vi "Main.vi"() -> ()   [LabVIEW 2024]
uses:
  1. CTL/Brain_Loop_CTL.ctl
  <vilib>/Utility/miscctls.llb/LVPointTypeDef.ctl
  <vilib>/Utility/sysdir.llb/System Directory Type.ctl
panel:
  in  "Python 경로":path=path "D:/Python39-32/python.exe"
  in  "모듈 경로":path=path "C:/Users/user/Desktop/CATS_V3.0/5. Python/Generate_map.py"
  in  "Subscribe_모듈 경로":path=path "C:/Users/user/Desktop/CATS_V3.0/5. Python/Mqtt_Subscribe_Client.py"
  in  "Publish_모듈 경로_2":path=path "C:/Users/user/Desktop/CATS_V3.0/5. Python/Mqtt_Publish_Client.py"
  in  "Publish_모듈 경로":path=path "C:/Users/user/Desktop/CATS_V3.0/5. Python/Mqtt_Publish_Client.py"
  out "2_3_Station_Averange_SoundSpeed_Chart":dbl(graph)
  out "Water_Velocity_Chart":dbl(graph)
  in  "거리":dbl=3750.0 format="%#_13g"
  in  "유속 데이터":T1
  in  "데이터 통계":T2
  in  "관리자":T3
  out "TX_그래프 5":bool
  out "RX_그래프 5":bool
  out "TX_LED_4":bool
  out "RX_LED_4":bool
  out "TX_그래프":bool
  out "RX_그래프":bool
  out "Station_5":i32[](graph)
  out "Station_4":i32[](graph)
  out "Station_1":i32[](graph)
  out "C":dbl
  out "3_Station_Index":i32
  out "2_Station_Index":i32
  out "반환값":string
  in  "전체메뉴_탭_컨트롤":enum32{"지도", "데이터 통계", "관리자", "유속 데이터"}(tab)=enum."데이터 통계"
  out "Station_3_송신시작":string
  out "Station_2_송신시작":string
  out "Station_2":i32[](graph)
  out "Station_3":i32[](graph)
  out "TX_LED_2":bool
  out "RX_LED_2":bool
  out "TX_LED_3":bool
  out "RX_LED_3":bool
  in  "관리자_내부_탭_컨트롤":enum32{"실시간 현황", "Setting"}(tab) caption="탭 컨트롤 2"
  out "Station_현황_GPS":i32[](listbox)
  out "데이터 통계 현황_결과창":string
  out "Station_현황_TRX_Controller":i32[](listbox)
  out "적용_LED 2":bool
  in  "Wake_UP버튼":bool
  out "지도모듈_LED":bool
  in  "지도":T4
  in  "Order":i32=12
  in  "Q 값":i32=4
  out "적용_LED":bool
  in  "적용 버튼":bool
  in  "정지":bool
  out "시작일":string
  out "로그 기록":string
  out "2_3_Station_Averange_SoundSpeed":dbl
  out "Water_Velocity":dbl
  # "Costal Acoustic Tomography(Ver1.1)"
  # "데이터 통계 현황"
  # "Costal Acoustic Tomography Setting"
  # "Coastal_TMC_Set_Variable"
  # "Coastal_TMC_Map_Web"
  # "Sation_Wake_UP"
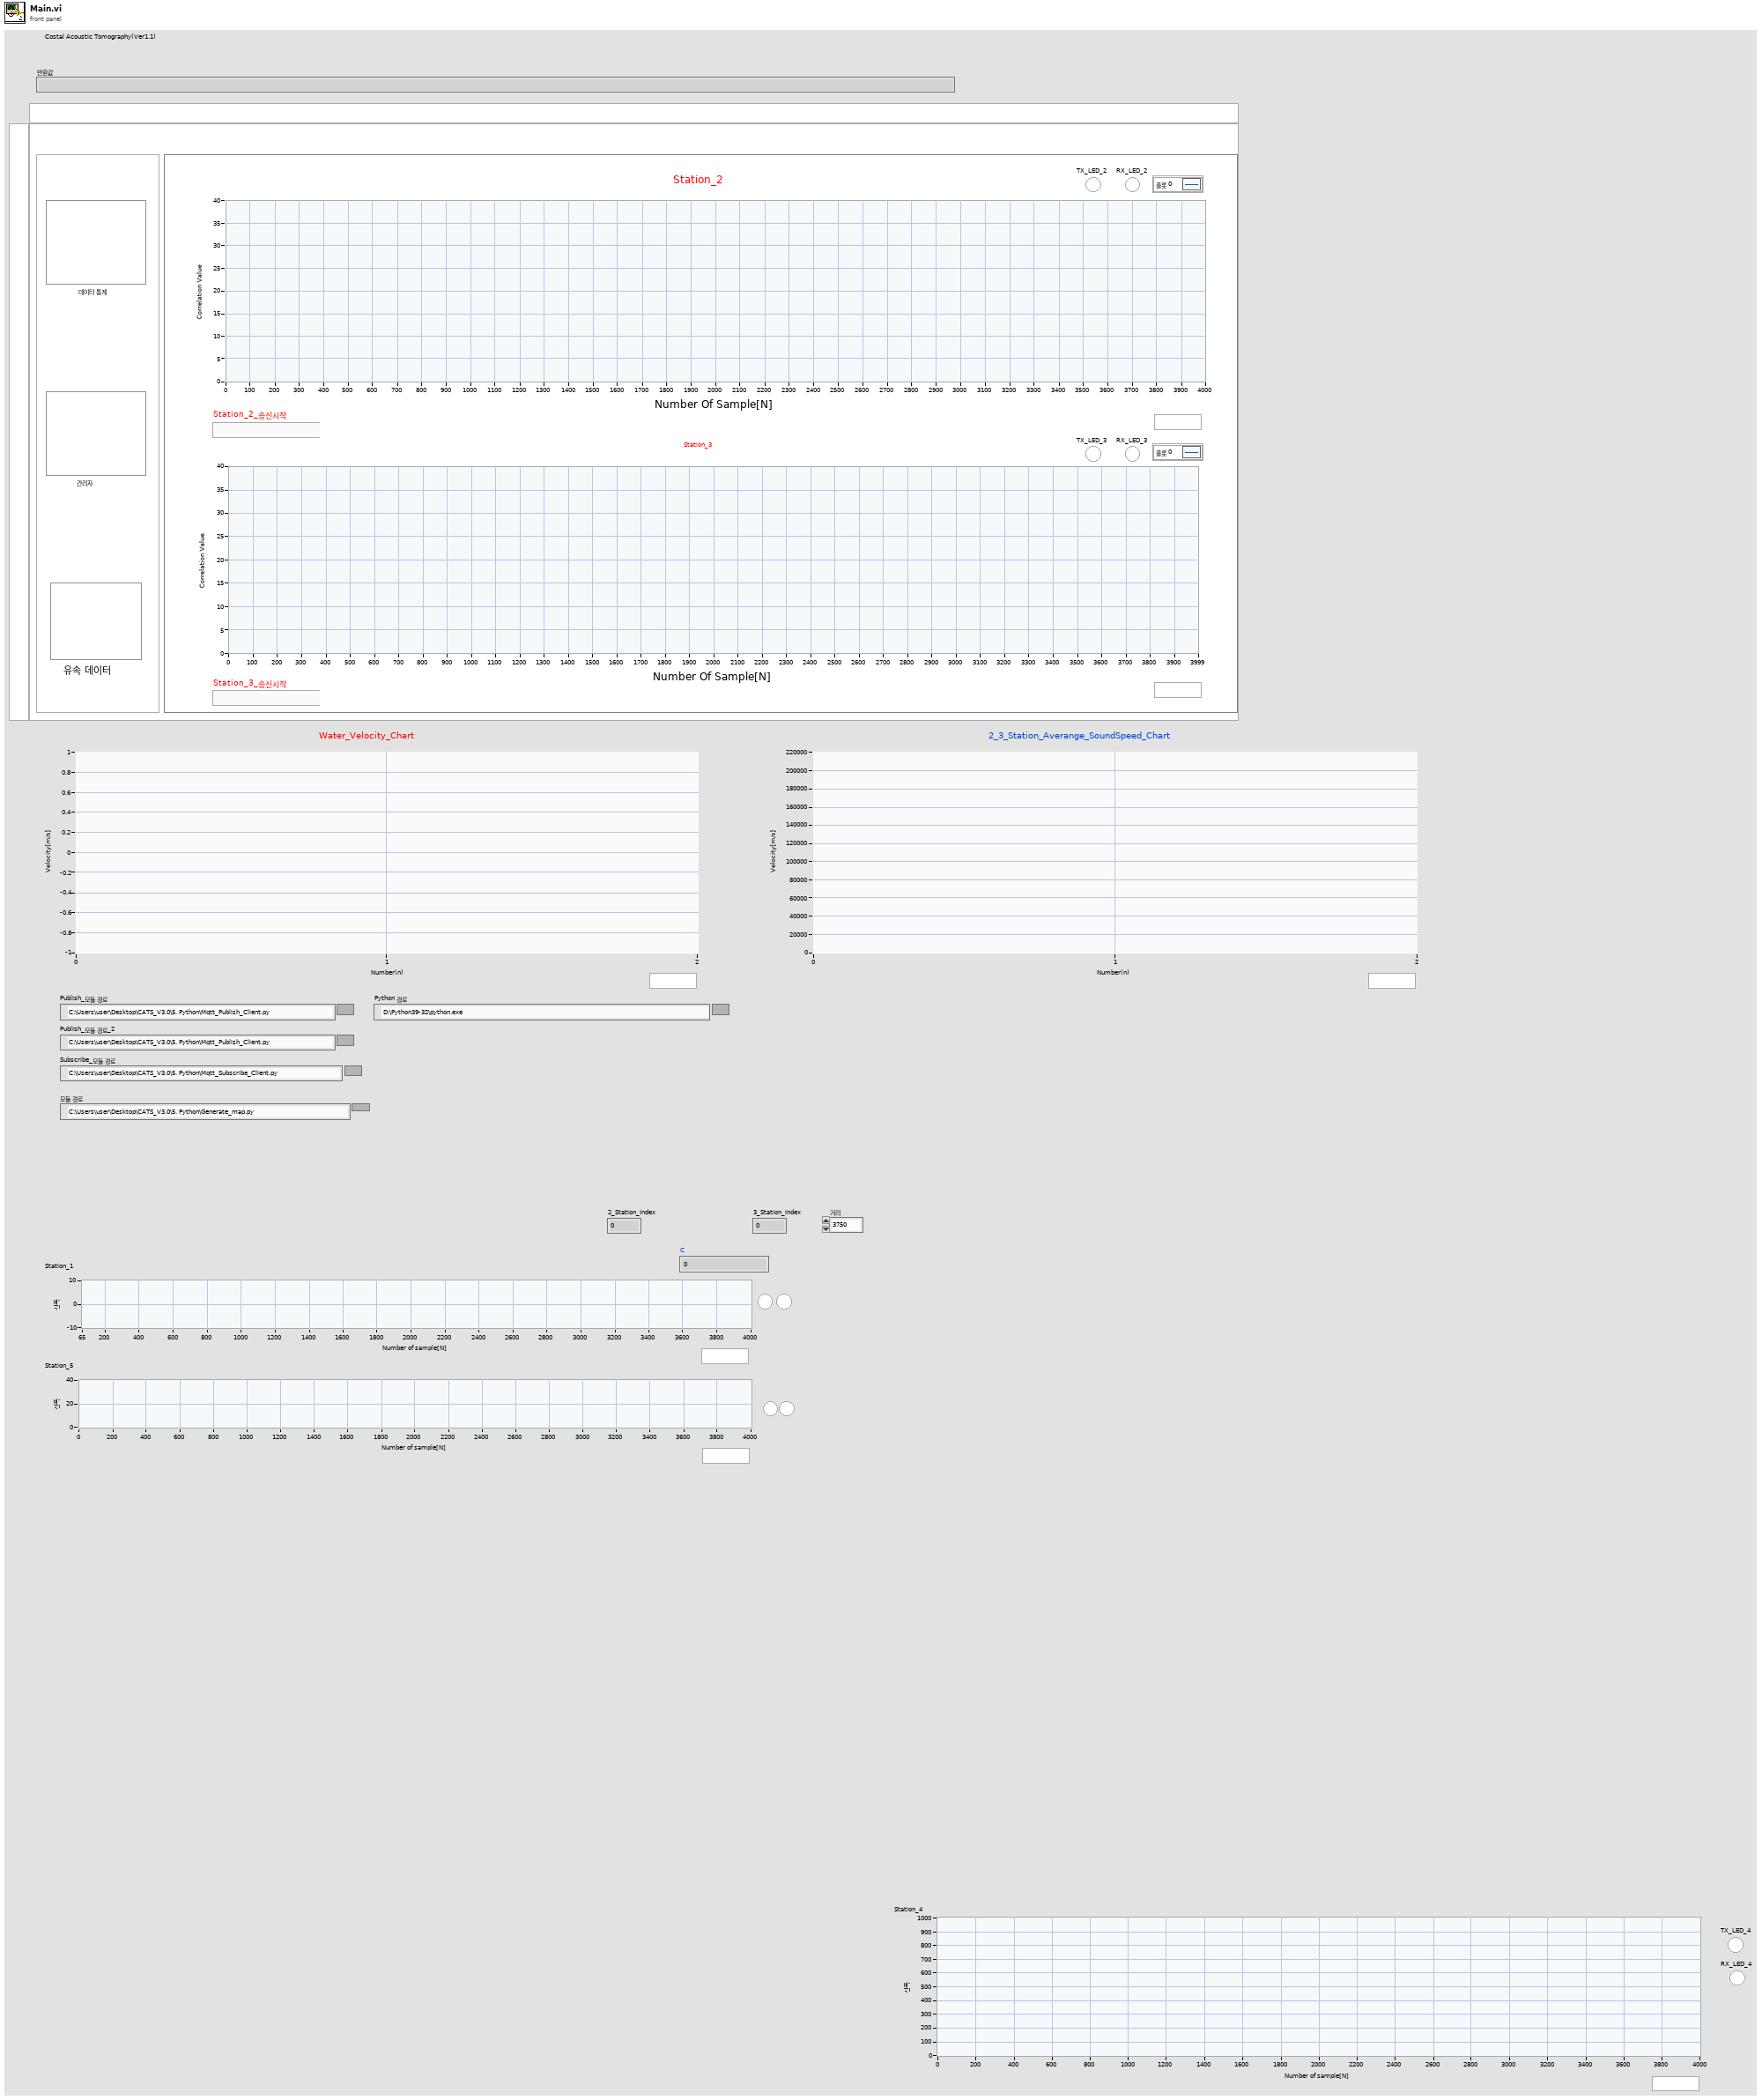
[diagram p1: front panel]
types:
  T1 = typedef "알림 컨트롤.ctl" = bool
  T2 = typedef "데이터 컨트롤.ctl" = bool
  T3 = typedef "관리 컨트롤.ctl" = bool
  T4 = typedef "지도 컨트롤.ctl" = bool
  T5 = cluster{"TX_그래프_LED":bool, "TX_그래프2_LED":bool, "TX_그래프3_LED":bool, "TX_그래프4_LED":bool, "TX_그래프5_LED":bool}
  T6 = cluster{"RX_그래프_LED":bool, "RX_그래프2_LED":bool, "RX_그래프3_LED":bool, "RX_그래프4_LED":bool, "RX_그래프5_LED":bool, "로그기록":string, "1_Station_Index":i32, "2_Station_Index":i32, "3_Station_Index":i32, "4_Station_Index":i32, "5_Station_Index":i32, "Velocity":dbl, "S_Flag":bool, "현재 날짜":string, "초기 날짜":string}
  T7 = typedef "Brain_Loop_CTL.ctl" = enum16{"초기화", "Mqtt_Subscribe", "Mqtt_Publish", "지도", "관리자", "데이터통계", "유속 데이터", "정지", "Mqtt_Publish_2"}
  T8 = typedef "LVPointTypeDef.ctl" = cluster{"Horizontal":i16, "Vertical":i16}
  T9 = typedef "System Directory Type.ctl" = i32
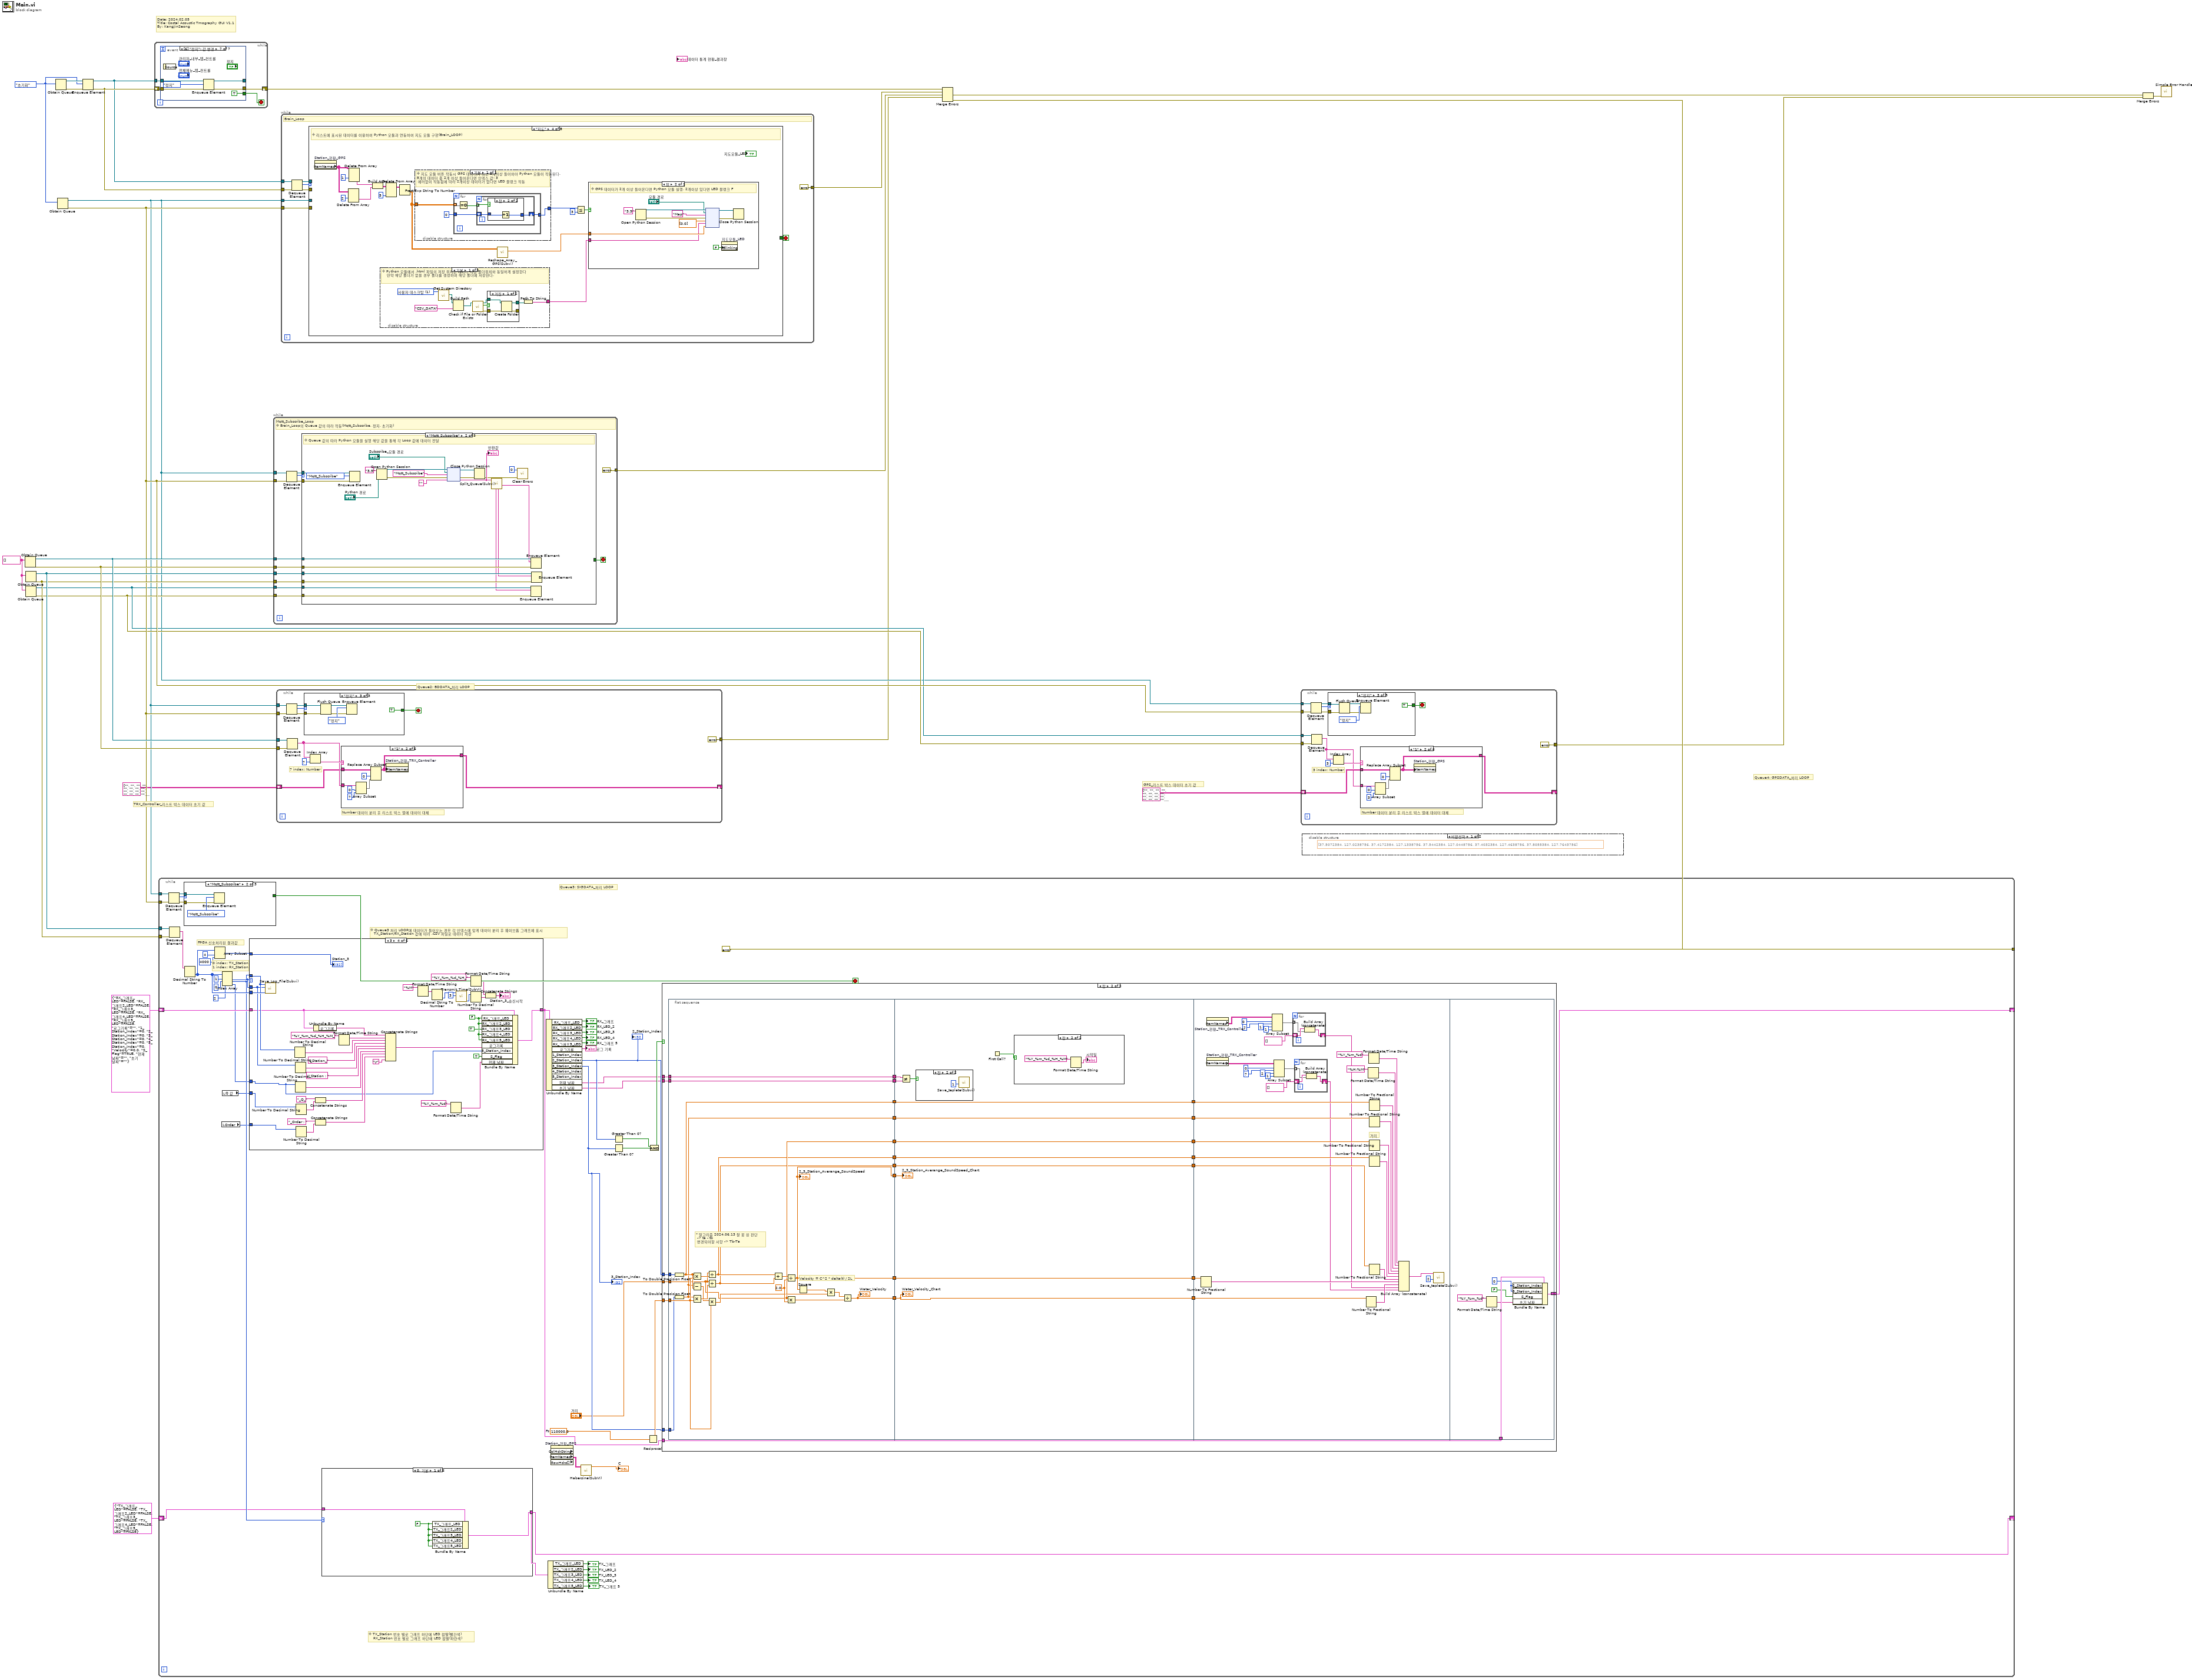
[diagram p0: block diagram]
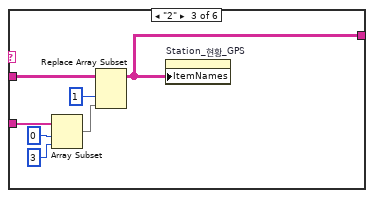
[diagram p4: hidden frame]
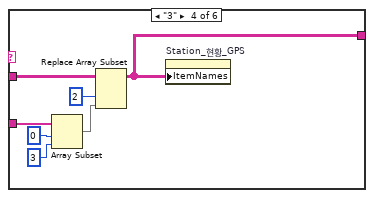
[diagram p5: hidden frame]
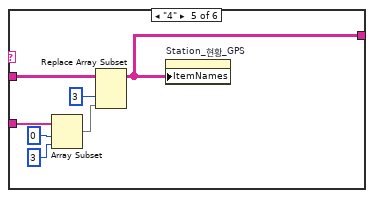
[diagram p6: hidden frame]
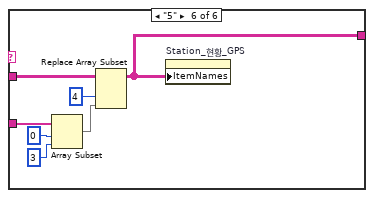
[diagram p7: hidden frame]
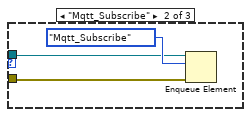
[diagram p9: hidden frame]
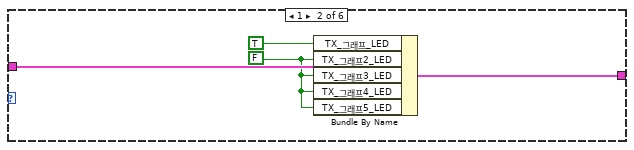
[diagram p13: hidden frame]
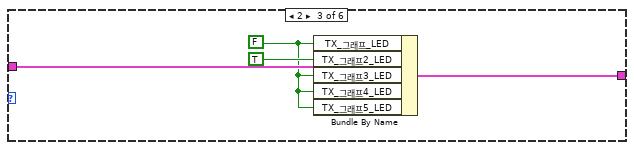
[diagram p14: hidden frame]
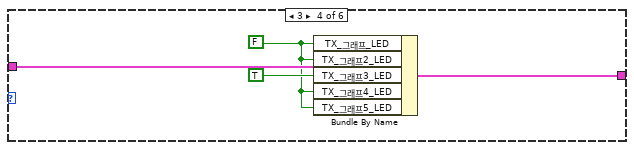
[diagram p15: hidden frame]
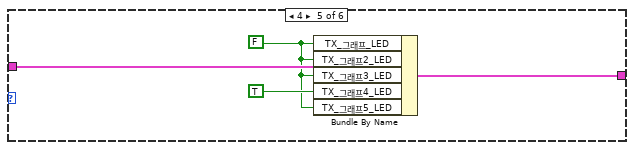
[diagram p16: hidden frame]
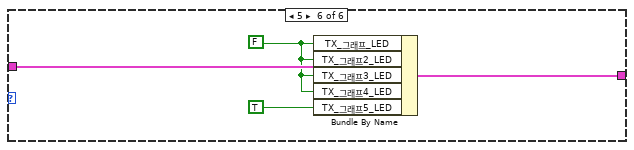
[diagram p17: hidden frame]
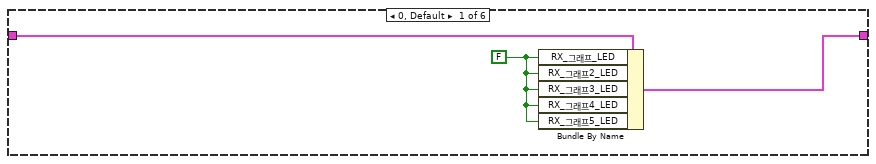
[diagram p18: hidden frame]
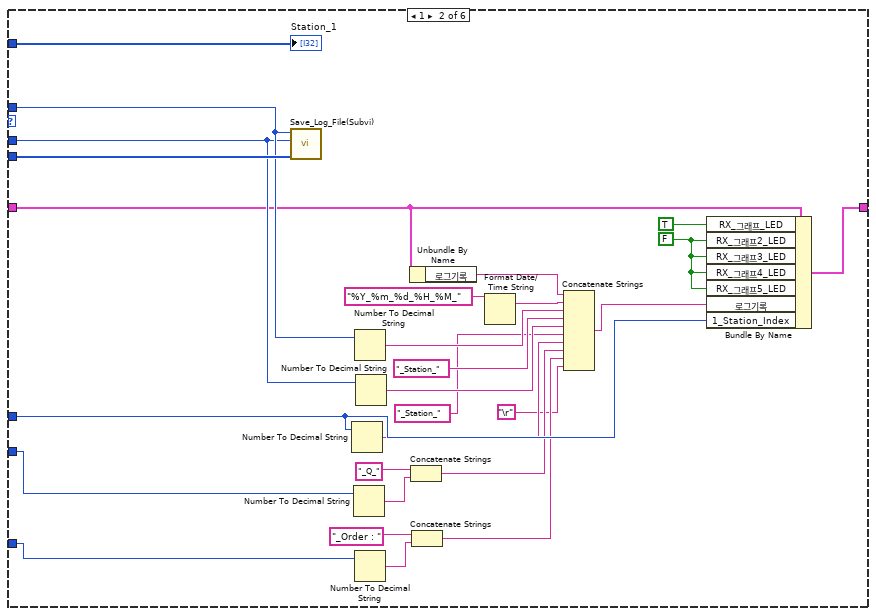
[diagram p19: hidden frame]
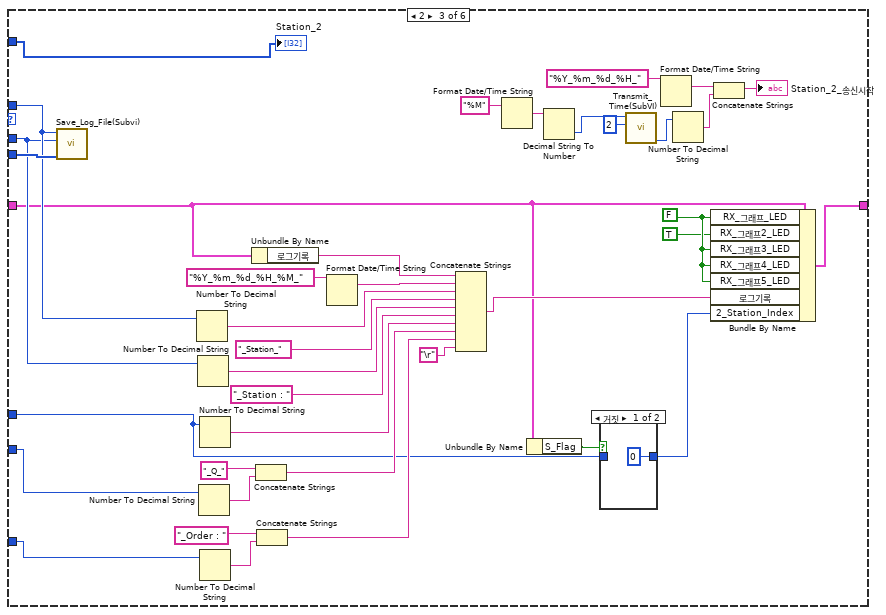
[diagram p20: hidden frame]
diagram:
  w20 = string[] []
  w21 = Brain_Loop_CTL."초기화"
  # "Queue2: BDDATA_처리 LOOP"
  # "Queue4: GPSDATA_처리 LOOP"
  # "GPS_리스트 박스 데이터 초기 값"
  # "TRX_Controller_리스트 박스 데이터 초기 값"
  # "Date: 2024.02.05\nTitle: Costal Acoustic Tmography GUI V1.1\nBy: KangJinSeong"
  n1 = Obtain Queue(element data type=w20) -> (queue out=w19:refnum<queue>, error out=w18:errorcluster)  [unwired: 4 in, 1 out]
  n2 = Obtain Queue(element data type=w20) -> (queue out=w17:refnum<queue>, error out=w16:errorcluster)  [unwired: 4 in, 1 out]
  n3 = Obtain Queue(element data type=w20) -> (queue out=w14:refnum<queue>, error out=w13:errorcluster)  [unwired: 4 in, 1 out]
  n4 = Obtain Queue(element data type=w21) -> (queue out=w24:refnum<queue>, error out=w26:errorcluster)  [unwired: 4 in, 1 out]
  n5 = Obtain Queue(element data type=w21) -> (queue out=w11:refnum<queue>, error out=w15:errorcluster)  [unwired: 4 in, 1 out]
  n6 = Enqueue Element(queue=w24, element=w21, error in (no error)=w26) -> (queue out=w12:refnum<queue>, error out=w25:errorcluster)  [unwired: 1 in, 1 out]
  n7 = while {
    tunnel: w12 -> [w29]
    shift-right: [w28] -> w23
    shift-left: w25 -> [w30]
    stop <- w27 stop-if-true
    n8 = event shown="[6] \"정지\": 값 변경" {
      selector: _ -> [_ _ _ _ _ _ _]
      dyn-events: _ -> [_ _ _ _ _ _ _]
      timeout: _ -> [_ _ _ _ _ _ _]
      tunnel: w30 -> [w35 w40 w42 w47 w55 w60 w66]
      tunnel: w29 -> [w34 w39 w44 w49 w54 w59 w65]
      tunnel: [w32 w37 w43 w48 w52 w58 w63] -> _
      tunnel: [w31 w36 w41 w46 w51 w57 w62] -> w28
      tunnel: [_ _ _ _ _ _ TRUE] -> w27
      event Value Change {
        n9 = event-data() -> ()  [unwired: 1 in, 1 out]
        n10 = Enqueue Element(queue=w34, element=Brain_Loop_CTL."지도", error in (no error)=w35) -> (queue out=w32:refnum<queue>, error out=w31:errorcluster)  [unwired: 1 in, 1 out]
      }
      event Value Change {
        n11 = event-data() -> ()  [unwired: 1 in, 1 out]
        n12 = Enqueue Element(queue=w39, element=Brain_Loop_CTL."데이터통계", error in (no error)=w40) -> (queue out=w37:refnum<queue>, error out=w36:errorcluster)  [unwired: 1 in, 1 out]
      }
      event "적용 버튼": Value Change {
        n13 = event-data() -> ()  [unwired: 1 in, 1 out]
        n14 = Enqueue Element(queue=w44, element=Brain_Loop_CTL."Mqtt_Publish", error in (no error)=w42) -> (queue out=w43:refnum<queue>, error out=w41:errorcluster)  [unwired: 1 in, 1 out]
      }
      event "Wake_UP버튼": Value Change {
        n15 = event-data() -> ()  [unwired: 1 in, 1 out]
        n16 = Enqueue Element(queue=w49, element=Brain_Loop_CTL."Mqtt_Publish_2", error in (no error)=w47) -> (queue out=w48:refnum<queue>, error out=w46:errorcluster)  [unwired: 1 in, 1 out]
      }
      event Value Change {
        n17 = event-data() -> ()  [unwired: 1 in, 1 out]
        n18 = Enqueue Element(queue=w54, element=Brain_Loop_CTL."관리자", error in (no error)=w55) -> (queue out=w52:refnum<queue>, error out=w51:errorcluster)  [unwired: 1 in, 1 out]
      }
      event Value Change {
        n19 = event-data() -> ()  [unwired: 1 in, 1 out]
        n20 = Enqueue Element(queue=w59, element=Brain_Loop_CTL."유속 데이터", error in (no error)=w60) -> (queue out=w58:refnum<queue>, error out=w57:errorcluster)  [unwired: 1 in, 1 out]
      }
      event "정지": Value Change {
        n21 = event-data() -> ()  [unwired: 1 in, 1 out]
        n22 = Enqueue Element(queue=w65, element=Brain_Loop_CTL."정지", error in (no error)=w66) -> (queue out=w63:refnum<queue>, error out=w62:errorcluster)  [unwired: 1 in, 1 out]
      }
    }
  }
  n23 = while {
    tunnel: w11 -> [w116]
    tunnel: w15 -> [w115]
    tunnel: w17 -> [w112]
    tunnel: w16 -> [w111]
    shift-right: [w76] -> _
    shift-left: T6 {"RX_그래프_LED"=FALSE, "RX_그래프2_LED"=FALSE, "RX_그래프3_LED"=FALSE, "RX_그래프4_LED"=FALSE, "RX_그래프5_LED"=FALSE, "로그기록"="", "1_Station_Index"=0, "2_Station_Index"=0, "3_Station_Index"=0, "4_Station_Index"=0, "5_Station_Index"=0, "Velocity"=0.0, "S_Flag"=TRUE, "현재 날짜"="", "초기 날짜"=""} -> [w100]
    shift-right: [w92] -> _
    shift-left: T5 {"TX_그래프_LED"=FALSE, "TX_그래프2_LED"=FALSE, "TX_그래프3_LED"=FALSE, "TX_그래프4_LED"=FALSE, "TX_그래프5_LED"=FALSE} -> [w98]
    tunnel: [errorcluster {"status"=FALSE, "code"=0, "source"=""} ("에러 상수")] -> w4
    stop <- w113 stop-if-true
    w80 = 110000.0  # Fs
    # "※ TX_Station 번호 별로 그래프 하단에 LED 점멸(빨간색)\n    RX_Station 번호 별로 그래프 하단에 LED 점멸(파란색)"
    # "※ Queue3 처리 LOOP에 데이터가 들어오는 경우 각 인덱스에 맞게 데이터 분리 후 웨이브폼 그래프에 표시\n   TX_Station/RX_Station 값에 따라 .CSV 파일로 데이터 저장"
    # "0 index: TX_Station\n1 index: RX_Station"
    # "FPGA 신호처리된 결과값"
    # "Queue3: SIGDATA_처리 LOOP"
    n24 = Dequeue Element(queue=w116, error in (no error)=w115) -> (queue out=w110:refnum<queue>, element=w114:T7, error out=w109:errorcluster)  [unwired: 1 in, 1 out]
    n25 = Dequeue Element(queue=w112, error in (no error)=w111) -> (element=w101:string[])  [unwired: 1 in, 3 out]
    n26 = case shown="\"Mqtt_Subscribe\"" w114 {
      tunnel: [_ _ TRUE] -> w113
      tunnel: w110 -> [_ w413 w416]
      tunnel: w109 -> [_ w414 w417]
      frame "초기화", Default {
      }
      frame "Mqtt_Subscribe" {
        n27 = Enqueue Element(queue=w413, element=Brain_Loop_CTL."Mqtt_Subscribe", error in (no error)=w414) -> ()  [unwired: 1 in, 3 out]
      }
      frame "정지" {
        n28 = Flush Queue(queue=w416, error in (no error)=w417) -> (queue out=w419:refnum<queue>, error out=w418:errorcluster)  [unwired: 1 out]
        n29 = Enqueue Element(queue=w419, element=Brain_Loop_CTL."정지", error in (no error)=w418) -> ()  [unwired: 1 in, 3 out]
      }
    }
    n30 = Decimal String To Number(string=w101) -> (number=w102:i32[])  [unwired: 2 in, 1 out]
    n31 = Array Subset(array=w102, index=4 ("인덱스"), length=4000 ("길이")) -> (w105:i32[])
    n32 = local read "Order"() -> (w86:i32)
    n33 = Index Array(array=w102, index #1=1 ("인덱스"), index #2=0 ("인덱스"), index #3=2 ("인덱스")) -> (element #1=w104:i32, element #2=w99:i32, element #3=w89:i32)
    n34 = local read "Q 값"() -> (w87:i32)
    n35 = case shown="3" w104 {
      tunnel: w105 -> [_ w279 w280 w320 w385 w412]
      tunnel: w99 -> [_ w276 w315 w356 w382 w409]
      tunnel: w104 -> [_ w275 w314 w355 w381 w408]
      tunnel: w102 -> [_ w278 w317 w358 w384 w411]
      tunnel: w100 -> [w252 w254 w295 w335 w360 w387]
      tunnel: [w251 w277 w316 w357 w383 w410] -> w77
      tunnel: w89 -> [_ w272 w281 w321 w378 w405]
      tunnel: w87 -> [_ w274 w313 w354 w380 w407]
      tunnel: w86 -> [_ w273 w312 w353 w379 w406]
      frame 0, Default {
        w250 = FALSE
        n36 = Bundle By Name(cluster=w252, "RX_그래프_LED"=w250, "RX_그래프2_LED"=w250, "RX_그래프3_LED"=w250, "RX_그래프4_LED"=w250, "RX_그래프5_LED"=w250) -> (w251:T6)
      }
      frame 1 {
        w270 = FALSE
        n37 = call "Save_Log_File(Subvi).vi"("TX_Station"=w276, "RX_Station"=w275, "1D data"=w278) -> ()  [unwired: 7 in, 1 out]
        n38 = Number To Decimal String(number=w272) -> (decimal integer string=w258:string)  [unwired: 1 in]
        n39 = Number To Decimal String(number=w274) -> (decimal integer string=w261:string)  [unwired: 1 in]
        n40 = Number To Decimal String(number=w276) -> (decimal integer string=w268:string)  [unwired: 1 in]
        n41 = Number To Decimal String(number=w273) -> (decimal integer string=w260:string)  [unwired: 1 in]
        n42 = Number To Decimal String(number=w275) -> (decimal integer string=w267:string)  [unwired: 1 in]
        n43 = Unbundle By Name(w254) -> ("로그기록"=w269:string)
        n44 = Concatenate Strings("_Q_" ("시간 포맷 문자열 (%c)"), w261) -> (w257:string)
        n45 = Concatenate Strings("_Order : " ("시간 포맷 문자열 (%c)"), w260) -> (w256:string)
        n46 = Format Date/Time String(time format string (%c)="%Y_%m_%d_%H_%M_" ("시간 포맷 문자열 (%c)")) -> (date/time string=w253:string)  [unwired: 2 in]
        n47 = Concatenate Strings(w269, w253, w268, "_Station_" ("시간 포맷 문자열 (%c)"), w267, "_Station_" ("시간 포맷 문자열 (%c)"), w258, w257, w256, "\r") -> (w263:string)
        n48 = Bundle By Name(cluster=w254, "RX_그래프_LED"=TRUE, "RX_그래프2_LED"=w270, "RX_그래프3_LED"=w270, "RX_그래프4_LED"=w270, "RX_그래프5_LED"=w270, "로그기록"=w263, "1_Station_Index"=w272) -> (w277:T6)
        "Station_1" <- w279
      }
      frame 2 {
        w311 = FALSE
        n49 = call "Save_Log_File(Subvi).vi"("TX_Station"=w315, "RX_Station"=w314, "1D data"=w317) -> ()  [unwired: 7 in, 1 out]
        n50 = Number To Decimal String(number=w315) -> (decimal integer string=w309:string)  [unwired: 1 in]
        n51 = Number To Decimal String(number=w314) -> (decimal integer string=w307:string)  [unwired: 1 in]
        n52 = Number To Decimal String(number=w313) -> (decimal integer string=w301:string)  [unwired: 1 in]
        n53 = Number To Decimal String(number=w281) -> (decimal integer string=w305:string)  [unwired: 1 in]
        n54 = Number To Decimal String(number=w312) -> (decimal integer string=w300:string)  [unwired: 1 in]
        n55 = Unbundle By Name(w295) -> ("로그기록"=w310:string)
        n56 = Concatenate Strings("_Q_" ("시간 포맷 문자열 (%c)"), w301) -> (w298:string)
        n57 = Concatenate Strings("_Order : " ("시간 포맷 문자열 (%c)"), w300) -> (w297:string)
        n58 = Format Date/Time String(time format string (%c)="%Y_%m_%d_%H_%M_" ("시간 포맷 문자열 (%c)")) -> (date/time string=w292:string)  [unwired: 2 in]
        n59 = Concatenate Strings(w310, w292, w309, "_Station_" ("시간 포맷 문자열 (%c)"), w307, "_Station : " ("시간 포맷 문자열 (%c)"), w305, w298, w297, "\r") -> (w304:string)
        n60 = Format Date/Time String(time format string (%c)="%M" ("시간 포맷 문자열 (%c)")) -> (date/time string=w289:string)  [unwired: 2 in]
        n61 = Unbundle By Name(w295) -> ("S_Flag"=w294:bool)
        n62 = Decimal String To Number(string=w289) -> (number=w284:i32)  [unwired: 2 in, 1 out]
        n63 = case shown="거짓" w294 {
          tunnel: w281 -> [_ w319]
          tunnel: [0 ("문자열") w319] -> w293
          frame False {
          }
          frame True {
          }
        }
        n64 = call "Transmit_Time(SubVI).vi"("Number"=2, "분"=w284) -> ("강제 변환(x)"=w288:i32)  [unwired: 9 in]
        n65 = Format Date/Time String(time format string (%c)="%Y_%m_%d_%H_" ("시간 포맷 문자열 (%c)")) -> (date/time string=w287:string)  [unwired: 2 in]
        n66 = Number To Decimal String(number=w288) -> (decimal integer string=w286:string)  [unwired: 1 in]
        n67 = Bundle By Name(cluster=w295, "RX_그래프_LED"=w311, "RX_그래프2_LED"=TRUE, "RX_그래프3_LED"=w311, "RX_그래프4_LED"=w311, "RX_그래프5_LED"=w311, "로그기록"=w304, "2_Station_Index"=w293) -> (w316:T6)
        n68 = Concatenate Strings(w287, w286) -> (→"Station_2_송신시작":string)
        "Station_2" <- w280
      }
      frame 3 {
        w351 = FALSE
        n69 = call "Save_Log_File(Subvi).vi"("TX_Station"=w356, "RX_Station"=w355, "1D data"=w358) -> ()  [unwired: 7 in, 1 out]
        n70 = Number To Decimal String(number=w356) -> (decimal integer string=w348:string)  [unwired: 1 in]
        n71 = Number To Decimal String(number=w355) -> (decimal integer string=w346:string)  [unwired: 1 in]
        n72 = Number To Decimal String(number=w321) -> (decimal integer string=w344:string)  [unwired: 1 in]
        n73 = Number To Decimal String(number=w354) -> (decimal integer string=w341:string)  [unwired: 1 in]
        n74 = Number To Decimal String(number=w353) -> (decimal integer string=w340:string)  [unwired: 1 in]
        n75 = Unbundle By Name(w335) -> ("로그기록"=w349:string)
        n76 = Concatenate Strings("_Q_" ("시간 포맷 문자열 (%c)"), w341) -> (w338:string)
        n77 = Concatenate Strings("_Order : " ("시간 포맷 문자열 (%c)"), w340) -> (w337:string)
        n78 = Format Date/Time String(time format string (%c)="%Y_%m_%d_%H_%M_" ("시간 포맷 문자열 (%c)")) -> (date/time string=w333:string)  [unwired: 2 in]
        n79 = Concatenate Strings(w349, w333, w348, "_Station_" ("시간 포맷 문자열 (%c)"), w346, "_Station : " ("시간 포맷 문자열 (%c)"), w344, w338, w337, "\r") -> (w343:string)
        n80 = Format Date/Time String(time format string (%c)="%M" ("시간 포맷 문자열 (%c)")) -> (date/time string=w330:string)  [unwired: 2 in]
        n81 = Decimal String To Number(string=w330) -> (number=w326:i32)  [unwired: 2 in, 1 out]
        n82 = Format Date/Time String(time format string (%c)="%Y_%m_%d" ("시간 포맷 문자열 (%c)")) -> (date/time string=w322:string)  [unwired: 2 in]
        n83 = call "Transmit_Time(SubVI).vi"("Number"=3, "분"=w326) -> ("강제 변환(x)"=w329:i32)  [unwired: 9 in]
        n84 = Format Date/Time String(time format string (%c)="%Y_%m_%d_%H_" ("시간 포맷 문자열 (%c)")) -> (date/time string=w328:string)  [unwired: 2 in]
        n85 = Number To Decimal String(number=w329) -> (decimal integer string=w327:string)  [unwired: 1 in]
        n86 = Bundle By Name(cluster=w335, "RX_그래프_LED"=w351, "RX_그래프2_LED"=w351, "RX_그래프3_LED"=TRUE, "RX_그래프4_LED"=w351, "RX_그래프5_LED"=w351, "로그기록"=w343, "3_Station_Index"=w321, "S_Flag"=TRUE, "현재 날짜"=w322) -> (w357:T6)
        n87 = Concatenate Strings(w328, w327) -> (→"Station_3_송신시작":string)
        "Station_3" <- w320
      }
      frame 4 {
        w376 = FALSE
        n88 = call "Save_Log_File(Subvi).vi"("TX_Station"=w382, "RX_Station"=w381, "1D data"=w384) -> ()  [unwired: 7 in, 1 out]
        n89 = Number To Decimal String(number=w378) -> (decimal integer string=w369:string)  [unwired: 1 in]
        n90 = Number To Decimal String(number=w380) -> (decimal integer string=w366:string)  [unwired: 1 in]
        n91 = Number To Decimal String(number=w382) -> (decimal integer string=w373:string)  [unwired: 1 in]
        n92 = Number To Decimal String(number=w379) -> (decimal integer string=w365:string)  [unwired: 1 in]
        n93 = Number To Decimal String(number=w381) -> (decimal integer string=w371:string)  [unwired: 1 in]
        n94 = Unbundle By Name(w360) -> ("로그기록"=w374:string)
        n95 = Concatenate Strings("_Q_" ("시간 포맷 문자열 (%c)"), w366) -> (w363:string)
        n96 = Concatenate Strings("_Order : " ("시간 포맷 문자열 (%c)"), w365) -> (w362:string)
        n97 = Format Date/Time String(time format string (%c)="%Y_%m_%d_%H_%M_" ("시간 포맷 문자열 (%c)")) -> (date/time string=w359:string)  [unwired: 2 in]
        n98 = Concatenate Strings(w374, w359, w373, "_Station_" ("시간 포맷 문자열 (%c)"), w371, "_Station : " ("시간 포맷 문자열 (%c)"), w369, w363, w362, "\r") -> (w368:string)
        n99 = Bundle By Name(cluster=w360, "RX_그래프_LED"=w376, "RX_그래프2_LED"=w376, "RX_그래프3_LED"=w376, "RX_그래프4_LED"=TRUE, "RX_그래프5_LED"=w376, "로그기록"=w368, "4_Station_Index"=w378) -> (w383:T6)
        "Station_4" <- w385
      }
      frame 5 {
        w403 = FALSE
        n100 = call "Save_Log_File(Subvi).vi"("TX_Station"=w409, "RX_Station"=w408, "1D data"=w411) -> ()  [unwired: 7 in, 1 out]
        n101 = Number To Decimal String(number=w409) -> (decimal integer string=w400:string)  [unwired: 1 in]
        n102 = Number To Decimal String(number=w408) -> (decimal integer string=w398:string)  [unwired: 1 in]
        n103 = Number To Decimal String(number=w407) -> (decimal integer string=w393:string)  [unwired: 1 in]
        n104 = Number To Decimal String(number=w406) -> (decimal integer string=w392:string)  [unwired: 1 in]
        n105 = Number To Decimal String(number=w405) -> (decimal integer string=w396:string)  [unwired: 1 in]
        n106 = Unbundle By Name(w387) -> ("로그기록"=w401:string)
        n107 = Concatenate Strings("_Q_" ("시간 포맷 문자열 (%c)"), w393) -> (w390:string)
        n108 = Concatenate Strings("_Order : " ("시간 포맷 문자열 (%c)"), w392) -> (w389:string)
        n109 = Format Date/Time String(time format string (%c)="%Y_%m_%d_%H_%M_" ("시간 포맷 문자열 (%c)")) -> (date/time string=w386:string)  [unwired: 2 in]
        n110 = Concatenate Strings(w401, w386, w400, "_Station_" ("시간 포맷 문자열 (%c)"), w398, "_Station : " ("시간 포맷 문자열 (%c)"), w396, w390, w389, "\r") -> (w395:string)
        n111 = Bundle By Name(cluster=w387, "RX_그래프_LED"=w403, "RX_그래프2_LED"=w403, "RX_그래프3_LED"=w403, "RX_그래프4_LED"=w403, "RX_그래프5_LED"=TRUE, "로그기록"=w395, "5_Station_Index"=w405) -> (w410:T6)
        "Station_5" <- w412
      }
    }
    n112 = case shown="0, 기본" w99 {
      tunnel: w98 -> [w229 w233 w237 w241 w245 w249]
      tunnel: [w228 w230 w236 w240 w244 w248] -> w92
      frame 0, Default {
        w227 = FALSE
        n113 = Bundle By Name(cluster=w229, "TX_그래프_LED"=w227, "TX_그래프2_LED"=w227, "TX_그래프3_LED"=w227, "TX_그래프4_LED"=w227, "TX_그래프5_LED"=w227) -> (w228:T5)
      }
      frame 1 {
        w231 = FALSE
        n114 = Bundle By Name(cluster=w233, "TX_그래프_LED"=TRUE, "TX_그래프2_LED"=w231, "TX_그래프3_LED"=w231, "TX_그래프4_LED"=w231, "TX_그래프5_LED"=w231) -> (w230:T5)
      }
      frame 2 {
        w234 = FALSE
        n115 = Bundle By Name(cluster=w237, "TX_그래프_LED"=w234, "TX_그래프2_LED"=TRUE, "TX_그래프3_LED"=w234, "TX_그래프4_LED"=w234, "TX_그래프5_LED"=w234) -> (w236:T5)
      }
      frame 3 {
        w238 = FALSE
        n116 = Bundle By Name(cluster=w241, "TX_그래프_LED"=w238, "TX_그래프2_LED"=w238, "TX_그래프3_LED"=TRUE, "TX_그래프4_LED"=w238, "TX_그래프5_LED"=w238) -> (w240:T5)
      }
      frame 4 {
        w242 = FALSE
        n117 = Bundle By Name(cluster=w245, "TX_그래프_LED"=w242, "TX_그래프2_LED"=w242, "TX_그래프3_LED"=w242, "TX_그래프4_LED"=TRUE, "TX_그래프5_LED"=w242) -> (w244:T5)
      }
      frame 5 {
        w246 = FALSE
        n118 = Bundle By Name(cluster=w249, "TX_그래프_LED"=w246, "TX_그래프2_LED"=w246, "TX_그래프3_LED"=w246, "TX_그래프4_LED"=w246, "TX_그래프5_LED"=TRUE) -> (w248:T5)
      }
    }
    n119 = Unbundle By Name(w77) -> ("RX_그래프_LED"=→"RX_그래프":bool, "RX_그래프2_LED"=→"RX_LED_2":bool, "RX_그래프3_LED"=→"RX_LED_3":bool, "RX_그래프4_LED"=→"RX_LED_4":bool, "RX_그래프5_LED"=→"RX_그래프 5":bool, "로그기록"=→"로그 기록":string, "2_Station_Index"=w73:i32, "3_Station_Index"=w72:i32, "현재 날짜"=w70:string, "초기 날짜"=w69:string)  [unwired: 3 out]
    "2_Station_Index" <- w73
    "3_Station_Index" <- w72
    n120 = Unbundle By Name(w92) -> ("TX_그래프_LED"=→"TX_그래프":bool, "TX_그래프2_LED"=→"TX_LED_2":bool, "TX_그래프3_LED"=→"TX_LED_3":bool, "TX_그래프4_LED"=→"TX_LED_4":bool, "TX_그래프5_LED"=→"TX_그래프 5":bool)
    n121 = property on="Station_현황_GPS" class="MCListbox (엄격한)" props=["ColHdrString", "ItemNames", "RowHdrs[]"]() -> ("ItemNames"=w71:string[][])  [unwired: 2 in, 4 out]
    n122 = call "Habersine(SubVI).vi"("아이템 이름"=w71) -> ("distance[m]"=→"C":dbl)  [unwired: 10 in]
    n123 = Greater Than 0?(x=w73) -> (x > 0?=w75:bool)
    n124 = Greater Than 0?(x=w72) -> (x > 0?=w74:bool)
    n125 = Reciprocal(x=w80) -> (1/x=w78:dbl)
    n126 = And(x=w75, y=w74) -> (x .and. y?=w79:bool)
    n127 = case shown="참" w79 {
      tunnel: w78 -> [_ w141]
      tunnel: "거리" -> [_ w142]
      tunnel: w77 -> [w117 w123]
      tunnel: [w117 w122] -> w76
      tunnel: w73 -> [_ w139]
      tunnel: w72 -> [_ w138]
      tunnel: w70 -> [_ w121]
      tunnel: w69 -> [_ w119]
      frame False {
      }
      frame True {
        n128 = flat-sequence {
          tunnel: w142 -> [w148]
          tunnel: w141 -> [w158]
          tunnel: [w153] -> w140
          tunnel: w139 -> [w152]
          tunnel: w138 -> [w151]
          tunnel: [w145] -> w137
          tunnel: [w150] -> w136
          tunnel: [w149] -> w134
          tunnel: [w148] -> w132
          tunnel: [w147] -> w129
          tunnel: [w146] -> w128
          tunnel: [w145] -> w125
          tunnel: w121 -> [w144]
          tunnel: [w144] -> w120
          tunnel: w119 -> [w143]
          tunnel: [w143] -> w118
          tunnel: w140 -> [w166]
          tunnel: w137 -> [w165]
          tunnel: w136 -> [w175]
          tunnel: [w175] -> w135
          tunnel: w134 -> [w174]
          tunnel: [w174] -> w133
          tunnel: w132 -> [w173]
          tunnel: [w173] -> w131
          tunnel: [w172] -> w130
          tunnel: w129 -> [w172]
          tunnel: w128 -> [w171]
          tunnel: [w171] -> w127
          tunnel: [w170] -> w126
          tunnel: w125 -> [w170]
          tunnel: [w166] -> w124
          tunnel: w120 -> [w169]
          tunnel: w118 -> [w168]
          tunnel: w135 -> [w213]
          tunnel: w133 -> [w212]
          tunnel: w131 -> [w211]
          tunnel: w130 -> [w210]
          tunnel: w127 -> [w209]
          tunnel: w126 -> [w208]
          tunnel: w124 -> [w207]
          tunnel: w123 -> [w226]
          tunnel: [w223] -> w122
          frame #0 {
            w160 = 2.0 ("y")
            # "* 알고리즘 2024.06.13 잘 못 된 판단\n -> ta - tb\n 변경되야할 사항 -> Tb-Ta"
            # "Velocity = C^2 * delta(t) / 2L"
            n129 = To Double Precision Float(number=w152) -> (double precision float=w150:dbl)
            n130 = To Double Precision Float(number=w151) -> (double precision float=w149:dbl)
            n131 = Multiply(x=w150, y=w158) -> (x*y=w163:dbl)
            n132 = Subtract(x=w149, y=w150) -> (x-y=w159:dbl)
            n133 = Multiply(x=w149, y=w158) -> (x*y=w162:dbl)
            n134 = Divide(x=w148, y=w163) -> (x/y=w147:dbl)
            n135 = Divide(x=w148, y=w162) -> (x/y=w146:dbl)
            n136 = Multiply(x=w159, y=w158) -> (x*y=w156:dbl)
            n137 = Add(x=w147, y=w146) -> (x+y=w161:dbl)
            n138 = Divide(x=w161, y=w160) -> (x/y=w145:dbl)
            "2_3_Station_Averange_SoundSpeed" <- w145
            n139 = Multiply(x=w148, y=w160) -> (x*y=w154:dbl)
            n140 = Square(x=w145) -> (x^2=w157:dbl)
            n141 = Multiply(x=w157, y=w156) -> (x*y=w155:dbl)
            n142 = Divide(x=w155, y=w154) -> (x/y=w153:dbl)
            "Water_Velocity" <- w153
          }
          frame #1 {
            n143 = Not Equal?(x=w169, y=w168) -> (x != y?=w167:bool)
            n144 = case shown="참" w167 {
              frame False {
              }
              frame True {
                n145 = call "Save_teplete(Subvi).vi"("숫자형"=1) -> ()  [unwired: 11 in]
              }
            }
            n146 = First Call?() -> (First Call?: T/F=w164:bool)
            n147 = case shown="참" w164 {
              frame False {
              }
              frame True {
                n148 = Format Date/Time String(time format string (%c)="%Y_%m_%d_%H_%M" ("시간 포맷 문자열 (%c)")) -> (date/time string=→"시작일":string)  [unwired: 2 in]
              }
            }
            "Water_Velocity_Chart" <- w166
            "2_3_Station_Averange_SoundSpeed_Chart" <- w165
          }
          frame #2 {
            # "거리"
            n149 = Number To Fractional String(number=w208) -> (F-format string=w197:string)  [unwired: 3 in]
            n150 = property on="Station_현황_TRX_Controller" class="MCListbox (엄격한)"() -> ("ItemNames"=w179:string[][])  [unwired: 2 in, 2 out]
            n151 = property on="Station_현황_TRX_Controller" class="MCListbox (엄격한)"() -> ("ItemNames"=w182:string[][])  [unwired: 2 in, 2 out]
            n152 = Array Subset(array=w179, index (row)=0 ("인덱스"), length (row)=7 ("길이"), index (col)=1 ("인덱스"), length (col)=1 ("길이")) -> (w187:string[][])
            n153 = Array Subset(array=w182, index (row)=0 ("인덱스"), length (row)=7 ("길이"), index (col)=2 ("인덱스"), length (col)=1 ("길이")) -> (w190:string[][])
            n154 = for {
              tunnel: w187 -> [w216] mode=indexing
              shift-right: [w215] -> w181
              shift-left: string[] [] -> [w217]
              n155 = Build Array (concatenate)(w217, w216) -> (w215:string[])
            }
            n156 = for {
              tunnel: w190 -> [w219] mode=indexing
              shift-right: [w218] -> w180
              shift-left: string[] [] -> [w220]
              n157 = Build Array (concatenate)(w220, w219) -> (w218:string[])
            }
            n158 = Number To Fractional String(number=w207) -> (F-format string=w196:string)  [unwired: 3 in]
            n159 = Format Date/Time String(time format string (%c)="%H:%M" ("시간 포맷 문자열 (%c)")) -> (date/time string=w193:string)  [unwired: 2 in]
            n160 = Format Date/Time String(time format string (%c)="%Y_%m_%d" ("시간 포맷 문자열 (%c)")) -> (date/time string=w203:string)  [unwired: 2 in]
            n161 = Number To Fractional String(number=w213) -> (F-format string=w202:string)  [unwired: 3 in]
            n162 = Number To Fractional String(number=w212) -> (F-format string=w201:string)  [unwired: 3 in]
            n163 = Number To Fractional String(number=w211) -> (F-format string=w200:string)  [unwired: 3 in]
            n164 = Number To Fractional String(number=w210) -> (F-format string=w199:string)  [unwired: 3 in]
            n165 = Number To Fractional String(number=w209) -> (F-format string=w198:string)  [unwired: 3 in]
            n166 = Build Array (concatenate)(w203, w193, w202, w201, w200, w199, w198, w197, w196, w181, w180) -> (w195:string[])
            n167 = call "Save_teplete(Subvi).vi"("숫자형"=2, "배열"=w195) -> ()  [unwired: 10 in]
          }
          frame #3 {
            w225 = 0 ("2_Station_Index")
            n168 = Format Date/Time String(time format string (%c)="%Y_%m_%d" ("시간 포맷 문자열 (%c)")) -> (date/time string=w221:string)  [unwired: 2 in]
            n169 = Bundle By Name(cluster=w226, "2_Station_Index"=w225, "3_Station_Index"=w225, "S_Flag"=FALSE, "초기 날짜"=w221) -> (w223:T6)
          }
        }
      }
    }
  }
  n170 = while {
    tunnel: w11 -> [w434]
    tunnel: w15 -> [w433]
    tunnel: w19 -> [w429]
    tunnel: w18 -> [w428]
    tunnel: [errorcluster {"status"=FALSE, "code"=0, "source"=""} ("에러 상수")] -> w6
    tunnel: w17 -> [w426]
    tunnel: w16 -> [w425]
    tunnel: w14 -> [w424]
    tunnel: w13 -> [w423]
    stop <- w432 stop-if-true
    # "Mqtt_Subscribe_Loop\n※ Brain_Loop의 Queue 값의 따라 작동(Mqtt_Subscribe, 정지, 초기화)"
    n171 = Dequeue Element(queue=w434, error in (no error)=w433) -> (queue out=w431:refnum<queue>, element=w422:T7, error out=w430:errorcluster)  [unwired: 1 in, 1 out]
    n172 = case shown="\"Mqtt_Subscribe\"" w422 {
      tunnel: [_ _ TRUE] -> w432
      tunnel: w431 -> [_ w455 w463]
      tunnel: w430 -> [_ w454 w462]
      tunnel: w429 -> [_ w452 _]
      tunnel: w428 -> [_ w451 _]
      tunnel: w426 -> [_ w450 _]
      tunnel: w425 -> [_ w449 _]
      tunnel: w424 -> [_ w448 _]
      tunnel: w423 -> [_ w447 _]
      frame "초기화", Default {
      }
      frame "Mqtt_Subscribe" {
        # "※ Queue 값의 따라 Python 모듈을 실행 해당 값을 통해 각 Loop 값에 데이터 전달"
        n173 = Enqueue Element(queue=w455, element=Brain_Loop_CTL."Mqtt_Subscribe", error in (no error)=w454) -> ()  [unwired: 1 in, 3 out]
        n174 = Open Python Session(python version="3.9" ("Python 버전"), python path="Python 경로") -> (session out=w441:refnum<k35>, error out=w457:errorcluster)  [unwired: 1 in]
        n175 = node(w441, "Subscribe_모듈 경로", "Mqtt_Subscribe" ("함수 이름"), w457, "") -> (w443:refnum<k35>, w442:errorcluster, w438:string)  [unwired: 2 out]
        "반환값" <- w438
        n176 = Close Python Session(session in=w443, error in=w442) -> (11:w437:errorcluster)
        n177 = call "Split_Queue(Subvi).vi"("입력 문자열"=w438) -> ("Split_Queue2_Result"=w446:string[], "Split_Queue3_Result"=w445:string[], "Split_Queue4_Result"=w444:string[])  [unwired: 5 in, 3 out]
        n178 = call <vilib>:"Clear Errors.vi"("error in (no error)"=w437, "specific error code to clear (0: all)"=0) -> ()  [unwired: 4 in, 2 out]
        n179 = Enqueue Element(queue=w452, element=w446, error in (no error)=w451) -> ()  [unwired: 1 in, 3 out]
        n180 = Enqueue Element(queue=w448, element=w444, error in (no error)=w447) -> ()  [unwired: 1 in, 3 out]
        n181 = Enqueue Element(queue=w450, element=w445, error in (no error)=w449) -> ()  [unwired: 1 in, 3 out]
      }
      frame "정지" {
        # "※ Queue 값의 따라 정지 인경우 해당 큐를 비우고 정지 전달"
        n182 = Flush Queue(queue=w463, error in (no error)=w462) -> (queue out=w461:refnum<queue>, error out=w460:errorcluster)  [unwired: 1 out]
        n183 = Enqueue Element(queue=w461, element=Brain_Loop_CTL."정지", error in (no error)=w460) -> ()  [unwired: 1 in, 3 out]
      }
    }
  }
  n184 = while {
    tunnel: w11 -> [w478]
    tunnel: w15 -> [w477]
    tunnel: w19 -> [w474]
    tunnel: w18 -> [w473]
    shift-right: [w466] -> _
    shift-left: string[][] [["", "", "", "", "", ""], ["", "", "", "", "", ""], ["", "", "", "", "", ""], ["", "", "", "", "", ""], ["", "", "", "", "", ""], ["", "", "", "", "", ""], ["", "", "", "", "", ""], ["", "", "", "", "", "0"], ["", "", "", "", "", ""], ["", "", "", "", "", ""], ["", "", "", "", "", ""], ["", "", "", "", "", ""], ["", "", "", "", "", ""]] -> [w467]
    tunnel: [errorcluster {"status"=FALSE, "code"=0, "source"=""} ("에러 상수")] -> w5
    stop <- w475 stop-if-true
    # "Number 데이터 분리 후 리스트 박스 열에 데이터 대체"
    # "7 index: Number"
    n185 = Dequeue Element(queue=w478, error in (no error)=w477) -> (queue out=w472:refnum<queue>, element=w476:T7, error out=w471:errorcluster)  [unwired: 1 in, 1 out]
    n186 = Dequeue Element(queue=w474, error in (no error)=w473) -> (element=w468:string[])  [unwired: 1 in, 3 out]
    n187 = case shown="\"정지\"" w476 {
      tunnel: [_ _ TRUE] -> w475
      tunnel: w472 -> [_ w516 w521]
      tunnel: w471 -> [_ w515 w520]
      frame "초기화", Default {
      }
      frame "Mqtt_Subscribe" {
        n188 = Enqueue Element(queue=w516, element=Brain_Loop_CTL."Mqtt_Subscribe", error in (no error)=w515) -> ()  [unwired: 1 in, 3 out]
      }
      frame "정지" {
        n189 = Flush Queue(queue=w521, error in (no error)=w520) -> (queue out=w519:refnum<queue>, error out=w518:errorcluster)  [unwired: 1 out]
        n190 = Enqueue Element(queue=w519, element=Brain_Loop_CTL."정지", error in (no error)=w518) -> ()  [unwired: 1 in, 3 out]
      }
    }
    n191 = Index Array(array=w468, index=7 ("인덱스")) -> (element=w469:string)
    n192 = case shown="\"1\"" w469 {
      tunnel: w468 -> [_ w483 w490 w497 w504 w511]
      tunnel: w467 -> [w479 w486 w493 w500 w507 w514]
      tunnel: [w479 w484 w491 w498 w505 w512] -> w466
      frame "거짓", Default {
      }
      frame "1" {
        # "Number 데이터 분리 후 리스트 박스 열에 데이처 대체"
        n193 = Array Subset(array=w483, index=0 ("차원 크기"), length=7 ("차원 크기")) -> (w480:string[])
        n194 = Replace Array Subset(array=w486, new element=w480, index (col)=0 ("비활성화된 인덱스 (열)")) -> (w484:string[][])  [unwired: 1 in]
        n195 = property on="Station_현황_TRX_Controller" class="MCListbox (엄격한)"("ItemNames"=w484) -> ()  [unwired: 2 in, 2 out]
      }
      frame "2" {
        n196 = Array Subset(array=w490, index=0 ("차원 크기"), length=7 ("차원 크기")) -> (w487:string[])
        n197 = Replace Array Subset(array=w493, new element=w487, index (col)=1 ("비활성화된 인덱스 (열)")) -> (w491:string[][])  [unwired: 1 in]
        n198 = property on="Station_현황_TRX_Controller" class="MCListbox (엄격한)"("ItemNames"=w491) -> ()  [unwired: 2 in, 2 out]
      }
      frame "3" {
        n199 = Array Subset(array=w497, index=0 ("차원 크기"), length=7 ("차원 크기")) -> (w494:string[])
        n200 = Replace Array Subset(array=w500, new element=w494, index (col)=2 ("비활성화된 인덱스 (열)")) -> (w498:string[][])  [unwired: 1 in]
        n201 = property on="Station_현황_TRX_Controller" class="MCListbox (엄격한)"("ItemNames"=w498) -> ()  [unwired: 2 in, 2 out]
      }
      frame "4" {
        n202 = Array Subset(array=w504, index=0 ("차원 크기"), length=7 ("차원 크기")) -> (w501:string[])
        n203 = Replace Array Subset(array=w507, new element=w501, index (col)=3 ("비활성화된 인덱스 (열)")) -> (w505:string[][])  [unwired: 1 in]
        n204 = property on="Station_현황_TRX_Controller" class="MCListbox (엄격한)"("ItemNames"=w505) -> ()  [unwired: 2 in, 2 out]
      }
      frame "5" {
        n205 = Array Subset(array=w511, index=0 ("차원 크기"), length=7 ("차원 크기")) -> (w508:string[])
        n206 = Replace Array Subset(array=w514, new element=w508, index (col)=4 ("비활성화된 인덱스 (열)")) -> (w512:string[][])  [unwired: 1 in]
        n207 = property on="Station_현황_TRX_Controller" class="MCListbox (엄격한)"("ItemNames"=w512) -> ()  [unwired: 2 in, 2 out]
      }
    }
  }
  n208 = while {
    tunnel: w25 -> [w532]
    tunnel: w12 -> [w531]
    tunnel: [errorcluster {"status"=FALSE, "code"=0, "source"=""} ("에러 상수")] -> w22
    tunnel: w11 -> [w525]
    tunnel: w15 -> [w524]
    stop <- w528 stop-if-true
    # "Brain_Loop"
    n209 = Dequeue Element(queue=w531, error in (no error)=w532) -> (queue out=w527:refnum<queue>, element=w529:T7, error out=w526:errorcluster)  [unwired: 1 in, 1 out]
    n210 = case shown="\"지도\"" w529 {
      tunnel: [_ _ _ _ _ _ _ w627] -> w528
      tunnel: w527 -> [_ _ _ _ _ _ _ _]
      tunnel: w526 -> [_ _ _ _ _ _ _ _]
      tunnel: w525 -> [w544 _ _ _ _ _ _ w630]
      tunnel: w524 -> [w543 _ _ _ _ _ _ w629]
      frame "초기화", Default {
        w533 = ""
        w538 = string[] ["TMC_SET_1", "TMC_SET_2", "TMC_SET_3", "TMC_SET_4", "TMC_SET_5"]
        w539 = i32[] [] ("웨이브폼 그래프")
        # "배터리 전원, 소모전류, 컨트롤 온도, 수온, 압력, Roll, Pitch"
        # "※ 1) GUI가 실행 될때는 (0,0)에서 실행된다. 2) 탭 컨트롤은 데이터 통계로 초기화 한다. 3) 웨이브폼 그래프 값 초기화 4) Station_현황_GPS, TRX_Controller의 리스트 초기화(Brain_LOOP)"
        n211 = Enqueue Element(queue=w544, element=Brain_Loop_CTL."Mqtt_Subscribe", error in (no error)=w543) -> ()  [unwired: 1 in, 3 out]
        n212 = property on="구획" class="Pane"("Origin"=T8 {"Horizontal"=0, "Vertical"=0} ("원점")) -> ()  [unwired: 2 in, 2 out]
        n213 = local write "로그 기록"("") -> ()
        n214 = property on="Station_현황_TRX_Controller" class="MCListbox (엄격한)"("ColHdrString"=w538, "ItemNames"=string[][] [["", "", "", "", "", "", ""], ["", "", "", "", "", "", ""], ["", "", "", "", "", "", ""], ["", "", "", "", "", "", ""], ["", "", "", "", "", "", ""], ["", "", "", "", "", "", ""], ["", "", "", "", "", "", ""], ["", "", "", "", "", "0", ""], ["", "", "", "", "", "", ""], ["", "", "", "", "", "", ""], ["", "", "", "", "", "", ""], ["", "", "", "", "", "", ""], ["", "", "", "", "", "", ""], ["", "", "", "", "", "", ""]], "RowHdrs[]"=string[] ["배터리 전원", "소모전류", "수온", "압력", "ROLL", "PITCH", "컨트롤 온도", "", ""]) -> ()  [unwired: 2 in, 2 out]
        n215 = property on="Station_현황_GPS" class="MCListbox (엄격한)"("ColHdrString"=w538, "ItemNames"=string[][] [["", "", "", "", "", ""], ["", "", "", "", "", ""], ["", "", "", "", "", ""], ["", "", "", "", "", ""], ["", "", "", "", "", ""], ["", "", "", "", "", ""], ["", "", "", "", "", ""], ["", "", "", "", "", "0"]], "RowHdrs[]"=string[] ["1PPS", "Latitude", "Longitude"]) -> ()  [unwired: 2 in, 2 out]
        n216 = property on="전체메뉴_탭_컨트롤" class="TabCtl (엄격한)"("Value"=enum32{"지도", "데이터 통계", "관리자", "유속 데이터"}."데이터 통계" ("전체메뉴_탭_컨트롤")) -> ()  [unwired: 2 in, 2 out]
        n217 = property on="Station_1" class="WFGraph (엄격한)"("Value"=w539) -> ()  [unwired: 2 in, 2 out]
        n218 = property on="Station_2" class="WFGraph (엄격한)"("Value"=w539) -> ()  [unwired: 2 in, 2 out]
        n219 = property on="Station_3" class="WFGraph (엄격한)"("Value"=w539) -> ()  [unwired: 2 in, 2 out]
        n220 = property on="Station_4" class="WFGraph (엄격한)"("Value"=w539) -> ()  [unwired: 2 in, 2 out]
        n221 = property on="Station_5" class="WFGraph (엄격한)"("Value"=w539) -> ()  [unwired: 2 in, 2 out]
        n222 = property on="Station_3_송신시작" class="Str"("Value"=w533) -> ()  [unwired: 2 in, 2 out]
        n223 = property on="Station_2_송신시작" class="Str"("Value"=w533) -> ()  [unwired: 2 in, 2 out]
      }
      frame "Mqtt_Publish" {
        # "※ 적용 버튼을 클릭시 Brain_Loop에서 Mqtt_Publish Python 모듈 실행(Brain_LOOP)['Stop,Order,Q,'Start']"
        n224 = Open Python Session(python version="3.9" ("Python 버전")) -> (session out=w554:refnum<k35>, error out=w550:errorcluster)  [unwired: 2 in]
        n225 = flat-sequence {
          frame #0 {
            n226 = property on="적용_LED" class="Bool (엄격한)"("Blinking"=TRUE ("점멸")) -> ()  [unwired: 2 in, 2 out]
            n227 = Wait (ms)(milliseconds to wait=u32 2000 ("대기 시간 (ms)")) -> ()  [unwired: 1 out]
          }
          frame #1 {
            n228 = property on="적용_LED" class="Bool (엄격한)"("Blinking"=FALSE ("점멸")) -> ()  [unwired: 2 in, 2 out]
          }
        }
        n229 = node(w554, "Publish_모듈 경로", "Mqtt_Publish" ("함수 이름"), w550, " ", "Order", "Q 값") -> (w552:refnum<k35>, w553:errorcluster)  [unwired: 3 in, 2 out]
        n230 = Close Python Session(session in=w552, error in=w553) -> ()  [unwired: 1 out]
      }
      frame "Mqtt_Publish_2" {
        # "※ 적용 버튼을 클릭시 Brain_Loop에서 Mqtt_Publish Python 모듈 실행(Brain_LOOP)['Stop,Order,Q,'Start']"
        n231 = Open Python Session(python version="3.9" ("Python 버전")) -> (session out=w565:refnum<k35>, error out=w561:errorcluster)  [unwired: 2 in]
        n232 = flat-sequence {
          frame #0 {
            n233 = property on="적용_LED 2" class="Bool (엄격한)"("Blinking"=TRUE ("점멸")) -> ()  [unwired: 2 in, 2 out]
            n234 = Wait (ms)(milliseconds to wait=u32 2000 ("대기 시간 (ms)")) -> ()  [unwired: 1 out]
          }
          frame #1 {
            n235 = property on="적용_LED 2" class="Bool (엄격한)"("Blinking"=FALSE ("점멸")) -> ()  [unwired: 2 in, 2 out]
          }
        }
        n236 = node(w565, "Publish_모듈 경로_2", "Mqtt_Publish_2" ("함수 이름"), w561, " ") -> (w563:refnum<k35>, w564:errorcluster)  [unwired: 1 in, 2 out]
        n237 = Close Python Session(session in=w563, error in=w564) -> ()  [unwired: 1 out]
      }
      frame "지도" {
        # "※ 리스트에 표시된 데이터를 이용하여 Python 모듈과 연동하여 지도 모듈 구현(Brain_LOOP)"
        n238 = property on="Station_현황_GPS" class="MCListbox (엄격한)"() -> ("ItemNames"=w579:string[][])  [unwired: 2 in, 2 out]
        n239 = Delete From Array(array=w579, index (row)=2 ("인덱스 (행)")) -> (deleted portion=w580:string[])  [unwired: 2 in, 1 out]
        n240 = Delete From Array(array=w579, index (row)=1 ("인덱스 (행)")) -> (deleted portion=w581:string[])  [unwired: 2 in, 1 out]
        n241 = Build Array(w581, w580) -> (w577:string[][])
        n242 = disable-structure shown="기본" {
          disable-tunnel: [w584] -> w570
          frame Enabled {
            w585 = T9 1 items=["사용자 홈"=0, "사용자 데스크탑"=1, "사용자 문서"=2, "사용자 어플리케이션 데이터"=3, "사용자 환경"=4, "사용자 임시"=5, "퍼블릭 문서"=6, "퍼블릭 어플리케이션 데이터"=7, "퍼블릭 환경"=8, "퍼블릭 캐시"=13, "시스템 코어 라이브러리"=9, "시스템 설치된 라이브러리"=10, "어플리케이션 파일"=11, "부팅 볼륨 루트"=12] ("system directory type")
            # "※ Python 모듈에서 .html 파일의 저장 위치는 데이터 저장 폴더위치와 동일하게 설정한다\n    만약 해당 폴더가 없을 경우 폴더를 생성하여 해당 폴더에 저장한다."
            n243 = call <vilib>:"Get System Directory.vi"("system directory type"=w585) -> ("system directory"=w587:path)  [unwired: 10 in]
            n244 = Build Path(base path=w587, name or relative path="CSV_DATA") -> (appended path=w591:path)
            n245 = call <vilib>:"Check if File or Folder Exists.vi"("path"=w591) -> ("error out"=w590:errorcluster, "file or folder exists?"=w588:bool, "dup path"=w589:path)  [unwired: 8 in]
            n246 = case shown="거짓" w588 {
              tunnel: w589 -> [w596 w598]
              tunnel: w590 -> [w595 w597]
              tunnel: [w594 w598] -> w592
              tunnel: [w593 w597] -> _
              frame False {
                n247 = Create Folder(path (use dialog)=w596, error in=w595) -> (created path=w594:path, error out=w593:errorcluster)  [unwired: 1 in, 1 out]
              }
              frame True {
              }
            }
            n248 = Path To String(path=w592) -> (string=w584:string)
          }
        }
        n249 = Delete From Array(array=w577, index (col)=5 ("비활성화된 인덱스 (열)")) -> (array with subset deleted=w576:string[][])  [unwired: 2 in, 1 out]
        n250 = Fract/Exp String To Number(string=w576) -> (number=w572:dbl[][])  [unwired: 3 in, 1 out]
        n251 = disable-structure shown="기본" {
          disable-tunnel: [w601] -> w575
          disable-tunnel: w572 -> [w599]
          frame Enabled {
            # "※ 지도 모듈 버튼 작동시 GPS 데이터가 최소 2개이상 들어와야 Python 모듈이 작동된다. 5개의 데이터 중 2개 이상 들어온다면 인덱스 값: 3 \n 에러없이 작동됨에 따라 2개이상 데이터가 없다면 LED 블랭크 작동"
            n252 = for {
              tunnel: w599 -> [w605] mode=indexing
              tunnel: [w603] -> w601
              tunnel: 0 -> [w602]
              n253 = Equal To 0?(x=w605) -> (x = 0?=w604:bool[])
              n254 = for {
                tunnel: w604 -> [w608] mode=indexing
                shift-right: [w606] -> w603
                shift-left: w602 -> [w607]
                n255 = case shown="참" w608 {
                  tunnel: w607 -> [w609 w611]
                  tunnel: [w609 w610] -> w606
                  frame False {
                  }
                  frame True {
                    n256 = Increment(x=w611) -> (x+1=w610:i32)
                  }
                }
              }
            }
          }
        }
        n257 = call "Reshape_Array_GPS(Subvi).vi"("2차원_GPS_Data"=w572) -> ("1차원_GPS_Data"=w571:dbl[])  [unwired: 10 in]
        n258 = Less Or Equal?(x=w575, y=3) -> (x <= y?=w573:bool)
        n259 = case shown="참" w573 {
          tunnel: w571 -> [_ w614]
          tunnel: w570 -> [_ w613]
          frame False {
            # "※ 2개이상 없다면 LED 블랭크"
            n260 = property on="지도모듈_LED" class="Bool (엄격한)"("Blinking"=TRUE ("점멸")) -> ()  [unwired: 2 in, 2 out]
          }
          frame True {
            # "※ GPS 데이터가 2개 이상 들어온다면 Python 모듈 실행, 2개이상 있다면 LED 블랭크 F"
            n261 = Open Python Session(python version="3.9" ("Python 버전")) -> (session out=w618:refnum<k35>, error out=w622:errorcluster)  [unwired: 2 in]
            n262 = node(w618, "모듈 경로", "Map" ("함수 이름"), w622, dbl[] [0.0], w613, w614) -> (w620:refnum<k35>, w619:errorcluster)  [unwired: 3 in, 2 out]
            n263 = property on="지도모듈_LED" class="Bool (엄격한)"("Blinking"=FALSE ("점멸")) -> ()  [unwired: 2 in, 2 out]
            n264 = Close Python Session(session in=w620, error in=w619) -> ()  [unwired: 1 out]
          }
        }
      }
      frame "관리자" {
        # "※ 관리자 버튼 클릭시 탭 컨트롤을 관리자로 변경(Brain_LOOP)"
        n265 = property on="전체메뉴_탭_컨트롤" class="TabCtl (엄격한)"("Value"=enum32{"지도", "데이터 통계", "관리자", "유속 데이터"}."관리자" ("전체메뉴_탭_컨트롤")) -> ()  [unwired: 2 in, 2 out]
      }
      frame "데이터통계" {
        # "※ 데이터통계 버튼 클릭시 탭 컨트롤을 데이터 통계로 변경(Brain_LOOP)"
        n266 = property on="전체메뉴_탭_컨트롤" class="TabCtl (엄격한)"("Value"=enum32{"지도", "데이터 통계", "관리자", "유속 데이터"}."데이터 통계" ("전체메뉴_탭_컨트롤")) -> ()  [unwired: 2 in, 2 out]
      }
      frame "유속 데이터" {
        # "※ 알림 버튼 클릭시 탭 컨트롤을 알림으로 변경(Brain_LOOP)"
        n267 = property on="전체메뉴_탭_컨트롤" class="TabCtl (엄격한)"("Value"=enum32{"지도", "데이터 통계", "관리자", "유속 데이터"}."유속 데이터" ("전체메뉴_탭_컨트롤")) -> ()  [unwired: 2 in, 2 out]
      }
      frame "정지" {
        w627 = TRUE
        # "※ 정지 버튼 클릭시 탭 컨트롤을 관리자로 변경(Brain_LOOP), 정지 버튼 클릭시 GUI 종료"
        n268 = Enqueue Element(queue=w630, element=Brain_Loop_CTL."정지", error in (no error)=w629) -> ()  [unwired: 1 in, 3 out]
        n269 = Quit LabVIEW(quit? (T)=w627) -> ()
      }
    }
  }
  n270 = Merge Errors(w23, w22, w6, w5, w4) -> (w2:errorcluster)
  n271 = while {
    tunnel: w11 -> [w644]
    tunnel: w15 -> [w643]
    tunnel: w14 -> [w641]
    tunnel: w13 -> [w640]
    shift-right: [w633] -> _
    shift-left: string[][] [["", "", "", "", "", ""], ["", "", "", "", "", ""], ["", "", "", "", "", ""], ["", "", "", "", "", "0"], ["", "", "", "", "", ""], ["", "", "", "", "", ""], ["", "", "", "", "", ""], ["", "", "", "", "", "0"], ["", "", "", "", "", ""], ["", "", "", "", "", ""], ["", "", "", "", "", ""], ["", "", "", "", "", ""], ["", "", "", "", "", ""]] -> [w635]
    tunnel: [errorcluster {"status"=FALSE, "code"=0, "source"=""} ("에러 상수")] -> w3
    stop <- w642 stop-if-true
    # "Number 데이터 분리 후 리스트 박스 열에 데이터 대체"
    # "3 index: Number"
    n272 = Dequeue Element(queue=w644, error in (no error)=w643) -> (queue out=w639:refnum<queue>, element=w632:T7, error out=w638:errorcluster)  [unwired: 1 in, 1 out]
    n273 = Dequeue Element(queue=w641, error in (no error)=w640) -> (element=w634:string[])  [unwired: 1 in, 3 out]
    n274 = case shown="\"정지\"" w632 {
      tunnel: [_ _ TRUE] -> w642
      tunnel: w639 -> [_ w682 w687]
      tunnel: w638 -> [_ w681 w686]
      frame "초기화", Default {
      }
      frame "Mqtt_Subscribe" {
        n275 = Enqueue Element(queue=w682, element=Brain_Loop_CTL."Mqtt_Subscribe", error in (no error)=w681) -> ()  [unwired: 1 in, 3 out]
      }
      frame "정지" {
        n276 = Flush Queue(queue=w687, error in (no error)=w686) -> (queue out=w684:refnum<queue>, error out=w685:errorcluster)  [unwired: 1 out]
        n277 = Enqueue Element(queue=w684, element=Brain_Loop_CTL."정지", error in (no error)=w685) -> ()  [unwired: 1 in, 3 out]
      }
    }
    n278 = Index Array(array=w634, index=3 ("인덱스")) -> (element=w636:string)
    n279 = case shown="\"1\"" w636 {
      tunnel: w634 -> [_ w650 w657 w664 w671 w678]
      tunnel: w635 -> [w645 w652 w659 w666 w673 w680]
      tunnel: [w645 w646 w653 w660 w667 w674] -> w633
      frame "거짓", Default {
      }
      frame "1" {
        # "Number 데이터 분리 후 리스트 박스 열에 데이처 대체"
        n280 = Array Subset(array=w650, index=0 ("차원 크기"), length=3 ("차원 크기")) -> (w647:string[])
        n281 = Replace Array Subset(array=w652, new element=w647, index (col)=0 ("비활성화된 인덱스 (열)")) -> (w646:string[][])  [unwired: 1 in]
        n282 = property on="Station_현황_GPS" class="MCListbox (엄격한)"("ItemNames"=w646) -> ()  [unwired: 2 in, 2 out]
      }
      frame "2" {
        # "Number 데이터 분리 후 리스트 박스 열에 데이처 대체"
        n283 = Array Subset(array=w657, index=0 ("차원 크기"), length=3 ("차원 크기")) -> (w654:string[])
        n284 = Replace Array Subset(array=w659, new element=w654, index (col)=1 ("비활성화된 인덱스 (열)")) -> (w653:string[][])  [unwired: 1 in]
        n285 = property on="Station_현황_GPS" class="MCListbox (엄격한)"("ItemNames"=w653) -> ()  [unwired: 2 in, 2 out]
      }
      frame "3" {
        # "Number 데이터 분리 후 리스트 박스 열에 데이처 대체"
        n286 = Array Subset(array=w664, index=0 ("차원 크기"), length=3 ("차원 크기")) -> (w661:string[])
        n287 = Replace Array Subset(array=w666, new element=w661, index (col)=2 ("비활성화된 인덱스 (열)")) -> (w660:string[][])  [unwired: 1 in]
        n288 = property on="Station_현황_GPS" class="MCListbox (엄격한)"("ItemNames"=w660) -> ()  [unwired: 2 in, 2 out]
      }
      frame "4" {
        # "Number 데이터 분리 후 리스트 박스 열에 데이처 대체"
        n289 = Array Subset(array=w671, index=0 ("차원 크기"), length=3 ("차원 크기")) -> (w668:string[])
        n290 = Replace Array Subset(array=w673, new element=w668, index (col)=3 ("비활성화된 인덱스 (열)")) -> (w667:string[][])  [unwired: 1 in]
        n291 = property on="Station_현황_GPS" class="MCListbox (엄격한)"("ItemNames"=w667) -> ()  [unwired: 2 in, 2 out]
      }
      frame "5" {
        # "Number 데이터 분리 후 리스트 박스 열에 데이처 대체"
        n292 = Array Subset(array=w678, index=0 ("차원 크기"), length=3 ("차원 크기")) -> (w675:string[])
        n293 = Replace Array Subset(array=w680, new element=w675, index (col)=4 ("비활성화된 인덱스 (열)")) -> (w674:string[][])  [unwired: 1 in]
        n294 = property on="Station_현황_GPS" class="MCListbox (엄격한)"("ItemNames"=w674) -> ()  [unwired: 2 in, 2 out]
      }
    }
  }
  n295 = disable-structure shown="비활성화" {
    frame Disabled {
      (unwired) dbl[] [37.5072384, 127.0238756, 37.4172384, 127.1338756, 37.5442384, 127.0448756, 37.4032384, 127.4638756, 37.8055384, 127.7643756]
    }
    frame Enabled {
    }
  }
  n296 = Merge Errors(w2, w3) -> (w1:errorcluster)
  n297 = call <vilib>:"Simple Error Handler.vi"("error in (no error)"=w1) -> ()  [unwired: 4 in, 5 out]
